vi "Drive Immediate.vi"(7 "Description":string, 8 "Command Info In":T1, 9 "Deadband Value":dbl=0.01, 10 "Right Setpoint":dbl, 11 "Left Setpoint":dbl) -> (0 "Command Info Out":T1)   [LabVIEW 2019]
doc: "Often used for joystick control, this VI checks to see that the joystick axes are outside the deadband and updates the motors appropriately."
uses:
  <vilib>/Rock Robotics/WPI/Framework/Command Status Info.ctl
  <vilib>/Rock Robotics/WPI/Framework/Completion Status.ctl
  <vilib>/Rock Robotics/WPI/Framework/Completion Notifier.ctl
  Implementation/Drive Setpoints.ctl
  Implementation/Drive Operations.ctl
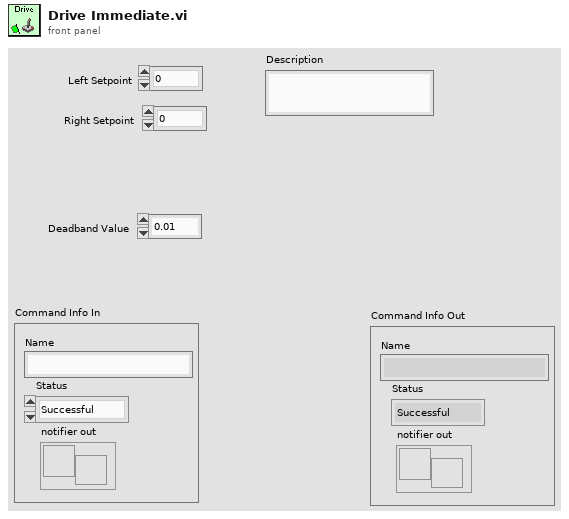
[diagram p1: front panel]
types:
  T1 = typedef "Command Status Info.ctl" = cluster{"Name":string, "Status":T2, "notifier out":T3}
  T2 = typedef "Completion Status.ctl" = enum16{"Successful", "Aborted", "Incomplete"}
  T3 = typedef "Completion Notifier.ctl" = refnum<notifier>
  T4 = typedef "Drive Setpoints.ctl" = cluster{"Operation":T5, "Left Setpoint":dbl, "Right Setpoint":dbl, "Duration":dbl, "Distance (inches)":dbl}
  T5 = typedef "Drive Operations.ctl" = enum16{"Reserve", "Read Current", "Immediate", "Drive for Time", "Drive for Distance"}
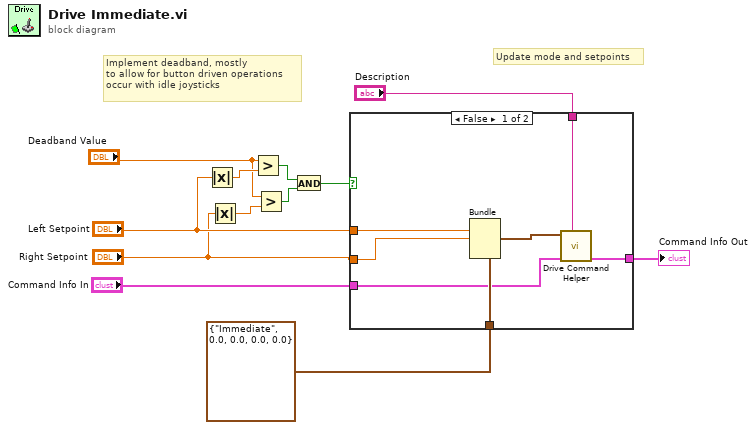
[diagram p0: block diagram]
diagram:
  # "Implement deadband, mostly\nto allow for button driven operations\noccur with idle joysticks"
  # "Update mode and setpoints"
  n1 = Absolute Value(x="Left Setpoint") -> (abs(x)=w12:dbl)
  n2 = Absolute Value(x="Right Setpoint") -> (abs(x)=w4:dbl)
  n3 = Greater?(x="Deadband Value", y=w12) -> (0:w6:bool)
  n4 = Greater?(x="Deadband Value", y=w4) -> (0:w2:bool)
  n5 = And(x=w6, y=w2) -> (x .and. y?=w5:bool)
  n6 = case shown="False" w5 {
    tunnel: "Left Setpoint" -> [w19 _]
    tunnel: T4 {"Operation"=enum."Immediate", "Left Setpoint"=0.0, "Right Setpoint"=0.0, "Duration"=0.0, "Distance (inches)"=0.0} ("SubSystem Data") -> [w18 _]
    tunnel: [w17 w20] -> w11
    tunnel: "Command Info In" -> [w16 w20]
    tunnel: "Description" -> [w15 _]
    tunnel: "Right Setpoint" -> [w14 _]
    frame False {
      n7 = Bundle(cluster=w18, "Left Setpoint"=w19, "Right Setpoint"=w14) -> (w13:T4)  [unwired: 3 in]
      n8 = call "Drive Command Helper.vi"("Description"=w15, "Command Info In"=w16, "SubSystem Data"=w13) -> ("Command Info Out"=w17:T1)  [unwired: 6 in, 2 out]
    }
    frame True {
    }
  }
  "Command Info Out" <- w11
